vi "Parse-line.vi"(6 "State data in":T1, 8 "error in":errorcluster, 10 "Line in":string, 11 "Elements in":refnum<class "Element-XML.lvclass">[](array[class])) -> (0 "error IO":errorcluster, 2 "Remaining line":string, 3 "Elements":refnum<class "Element-XML.lvclass">[](array[class]), 4 "State data":T1)   [LabVIEW 2013, in "HardwareCharacterization.lvlib" / "Element-XML.lvclass"]
uses:
  Element-XML.lvclass
  XML-parser-state.ctl
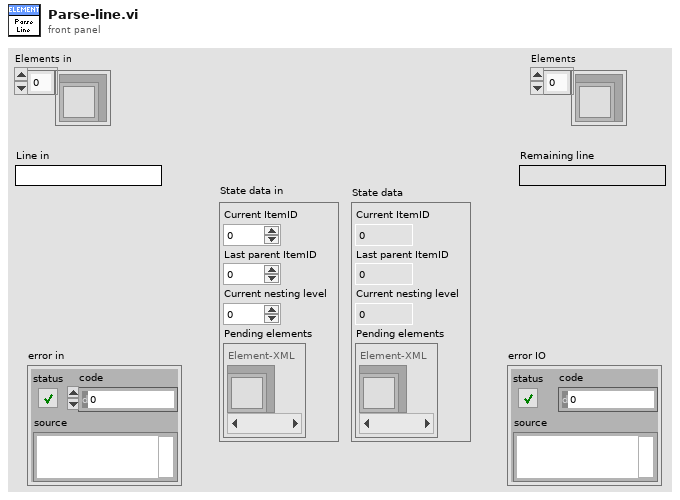
[diagram p1: front panel]
types:
  T1 = typedef "HardwareCharacterization.lvlib/Element-XML.lvclass/XML-parser-state.ctl" = cluster{"Current ItemID":u32, "Last parent ItemID":u32, "Current nesting level":i16, "Pending elements":refnum<class "Element-XML.lvclass">[]}
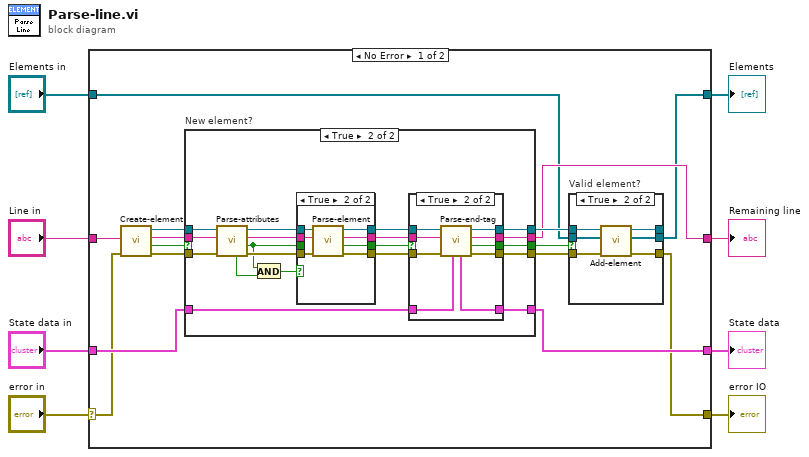
[diagram p0: block diagram]
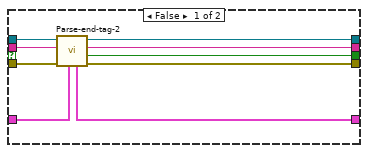
[diagram p3: hidden frame]
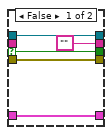
[diagram p4: hidden frame]
diagram:
  n1 = case shown="No Error" "error in" {
    selector: "error in" -> [w10 w89]
    tunnel: [w9 w89] -> w7
    tunnel: "Elements in" -> [w12 w88]
    tunnel: [w11 w88] -> w5
    tunnel: "Line in" -> [w23 w86]
    tunnel: "State data in" -> [w18 w87]
    tunnel: [w17 w87] -> w2
    tunnel: [w14 w86] -> w1
    frame No Error {
      n2 = call "Create-element.vi"("error in (no error)"=w10, "String in"=w23) -> ("error out"=w20:errorcluster, "Start tag?"=w19:bool, "Remaining string"=w21:string, "Element-XML out"=w22:refnum<class "Element-XML.lvclass">)  [unwired: 6 in]
      n3 = case "New element?" shown="True" w19 {
        tunnel: w22 -> [w41 w60]
        tunnel: w21 -> [w40 w59]
        tunnel: w20 -> [w35 w58]
        tunnel: [w36 w47] -> w13
        tunnel: [w38 w44] -> w16
        tunnel: [w39 w43] -> w14
        tunnel: [w37 w42] -> w15
        tunnel: w18 -> [w34 w46]
        tunnel: [w33 w45] -> w17
        frame False {
          n4 = call "Parse-end-tag-2.vi"("State data in"=w34, "error in (no error)"=w35, "String in"=w40, "Element-XML in"=w41) -> ("error out"=w36:errorcluster, "Valid element?"=w37:bool, "Remaining string"=w39:string, "Element-XML"=w38:refnum<class "Element-XML.lvclass">, "State data"=w33:T1)  [unwired: 3 in]
        }
        frame True {
          n5 = call-dynamic "Parse-attributes.vi"("error in (no error)"=w58, "String in"=w59, "Element-XML in"=w60) -> ("error out"=w53:errorcluster, "Valid attributes?"=w52:bool, "Remaining string"=w55:string, "Element-XML out"=w54:refnum<class "Element-XML.lvclass">, "Remaining content?"=w57:bool)  [unwired: 4 in]
          n6 = And(x=w52, y=w57) -> (x .and. y?=w56:bool)
          n7 = case shown="True" w56 {
            tunnel: [w75 w85] -> w48
            tunnel: [w78 w84] -> w51
            tunnel: [w77 w83] -> w50
            tunnel: [w76 w82] -> w49
            tunnel: w55 -> [w77 w81]
            tunnel: w54 -> [w78 w80]
            tunnel: w53 -> [w75 w79]
            tunnel: w52 -> [w76 _]
            frame False {
            }
            frame True {
              n8 = call-dynamic "Parse-element.vi"("error in (no error)"=w79, "String in"=w81, "Element-XML in"=w80) -> ("error out"=w85:errorcluster, "Valid element?"=w82:bool, "Remaining string"=w83:string, "Element-XML out"=w84:refnum<class "Element-XML.lvclass">)  [unwired: 5 in]
            }
          }
          n9 = case shown="True" w49 {
            selector: w49 -> [w62 _]
            tunnel: w51 -> [w63 w74]
            tunnel: w50 -> [_ w73]
            tunnel: w48 -> [w64 w72]
            tunnel: [w64 w71] -> w47
            tunnel: w46 -> [w65 w67]
            tunnel: [w65 w66] -> w45
            tunnel: [w63 w69] -> w44
            tunnel: ["" w70] -> w43
            tunnel: [w62 w68] -> w42
            frame False {
            }
            frame True {
              n10 = call-dynamic "Parse-end-tag.vi"("State data in"=w67, "error in (no error)"=w72, "String in"=w73, "Element-XML in"=w74) -> ("error out"=w71:errorcluster, "Valid element?"=w68:bool, "Remaining string"=w70:string, "Element-XML out"=w69:refnum<class "Element-XML.lvclass">, "State data"=w66:T1)  [unwired: 3 in]
            }
          }
        }
      }
      n11 = case "Valid element?" shown="True" w15 {
        tunnel: w16 -> [w26 w32]
        tunnel: w13 -> [w24 w31]
        tunnel: w12 -> [w25 w30]
        tunnel: [w25 w29] -> w11
        tunnel: [w26 w28] -> _
        tunnel: [w24 w27] -> w9
        frame False {
        }
        frame True {
          n12 = call "Add-element.vi"("error in (no error)"=w31, "Elements in"=w30, "Element-XML in"=w32) -> ("error out"=w27:errorcluster, "Elements"=w29:refnum<class "Element-XML.lvclass">[], "Element-XML out"=w28:refnum<class "Element-XML.lvclass">)  [unwired: 6 in]
        }
      }
    }
    frame Error {
    }
  }
  "Elements" <- w5
  "error IO" <- w7
  "State data" <- w2
  "Remaining line" <- w1
